vi "Power Monitor.vi"() -> ()   [LabVIEW 2013]
panel:
  out "SPEED - FPM":dbl format="%3.1f"
  out "DOWNFORCE":dbl format="%1.1f"
  out "TRACTIVE LOAD":dbl format="%1.1f"
  in  "Stop Button":bool
  out "Boolean 9":bool
  in  "Boolean 11":bool
  out "Boolean 8":bool
  in  "Boolean 10":bool
  out "Boolean 3":bool
  out "Boolean 2":bool
  in  "Boolean":bool
  out "DC AMPS":dbl format="%.3f"
  out "DC VOLTS":dbl format="%-2.1f"
  out "AC FREQUENCY":dbl format="%4.1f"
  out "AC AMPS L3":dbl format="%1.2f"
  out "AC VOLTS L3":dbl format="%3.1f"
  out "AC AMPS L2":dbl format="%1.2f"
  out "AC VOLTS L2":dbl format="%1.1f"
  out "AC AMPS L1":dbl format="%1.2f"
  out "AC VOLTS L1":dbl format="%1.1f"
  in  "DC V":dbl(slide) scale=0.0..30.0
  in  "DC A":dbl(slide) scale=0.0..5.0
  in  "AC FREQ":dbl(slide) scale=0.0..400.0
  in  "AC VOLTS":dbl(slide) scale=0.0..115.0
  in  "AC AMPS":dbl(slide) scale=0.0..25.0
  # "OPERATION"
  # "LOAD PARAMETERS"
  # "BRK"
  # "OFF"
  # "RUN"
  # "OFF"
  # "FWD"
  # "AFT"
  # "POWER CONSUMPTION"
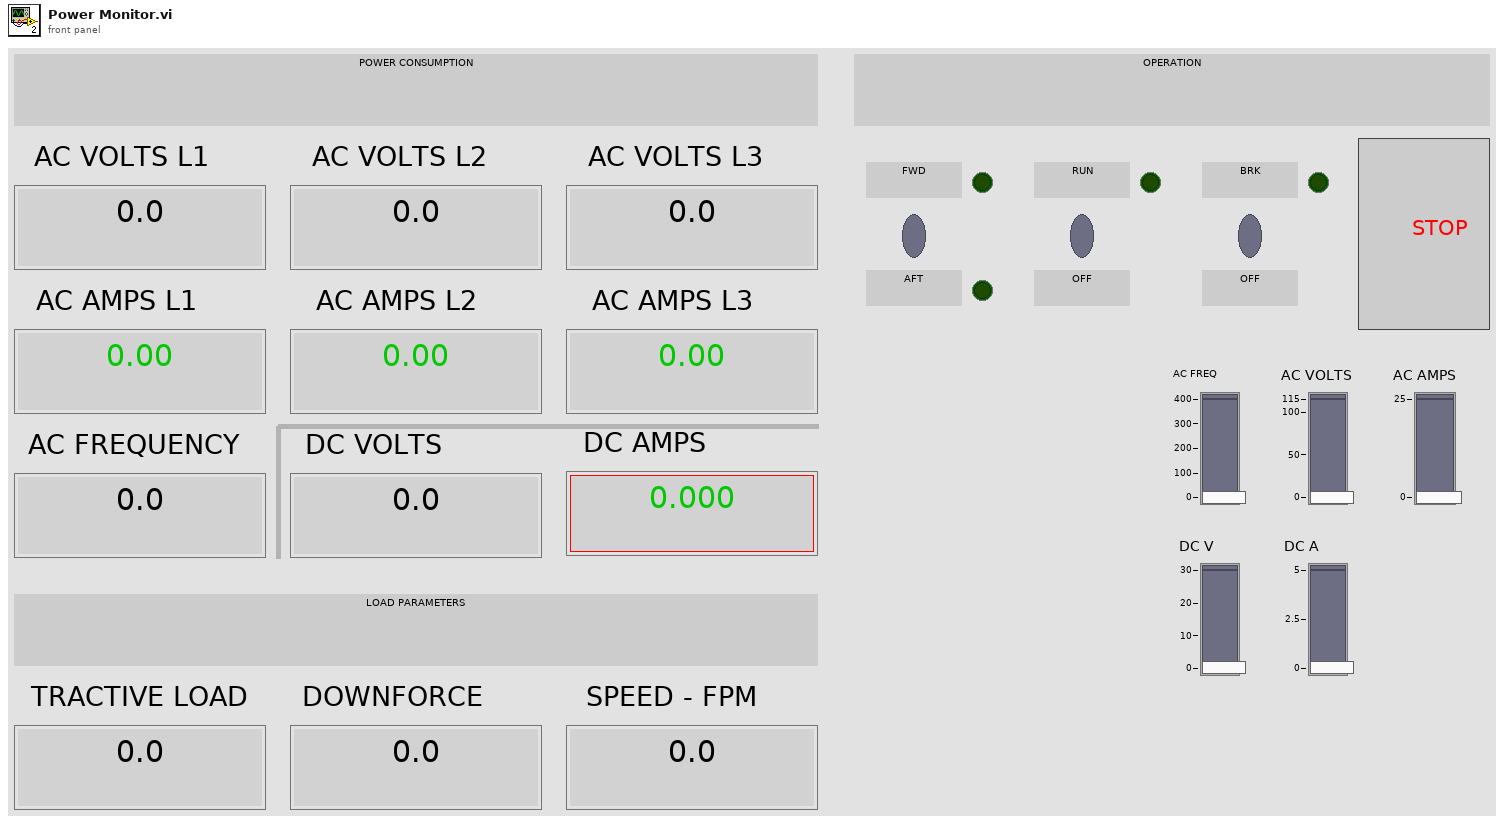
[diagram p1: front panel]
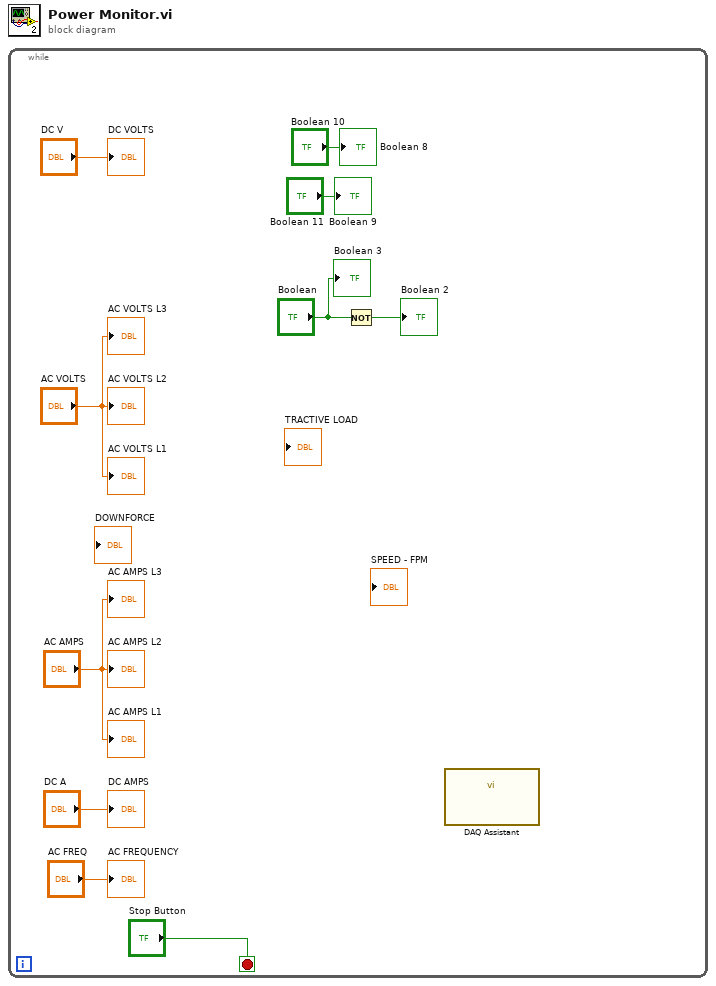
[diagram p0: block diagram]
diagram:
  n1 = while {
    stop <- "Stop Button" stop-if-true
    n2 = Not(x="Boolean") -> (.not. x?=→"Boolean 2":bool)
    n3 = call "DAQ Assistant"() -> ()  [unwired: 12 in]
    "DC VOLTS" <- "DC V"
    "DC AMPS" <- "DC A"
    "AC AMPS L1" <- "AC AMPS"
    "AC VOLTS L1" <- "AC VOLTS"
    "AC VOLTS L2" <- "AC VOLTS"
    "AC AMPS L2" <- "AC AMPS"
    "AC VOLTS L3" <- "AC VOLTS"
    "AC AMPS L3" <- "AC AMPS"
    "AC FREQUENCY" <- "AC FREQ"
    "Boolean 3" <- "Boolean"
    "Boolean 8" <- "Boolean 10"
    "Boolean 9" <- "Boolean 11"
  }
